vi "压力数据收集.vi"(10 "Value":dbl format="%_3g", 11 "数组in":dbl[][](array[numeric])) -> (1 "添加的数组":dbl[](array[numeric]), 2 "产品型号":string caption="型号字符串", 3 "数组out":dbl[][](array[numeric]))   [LabVIEW 2017]
panel:
  out "添加的数组 19":dbl[](array[numeric])
  out "MAX位置2":dbl
  out "添加的数组 20":dbl[](array[numeric])
  out "MAX位置1":dbl
  out "添加的数组 17":dbl[](array[numeric])
  out "MAX位置3":dbl
  out "添加的数组 18":dbl[](array[numeric])
  out "MAX位置18":dbl
  out "添加的数组 21":dbl[](array[numeric])
  out "MAX位置19":dbl
  out "添加的数组 14":dbl[](array[numeric])
  out "MAX位置17":dbl
  out "添加的数组 15":dbl[](array[numeric])
  out "MAX位置16":dbl
  out "添加的数组 16":dbl[](array[numeric])
  out "MAX位置15":dbl
  out "添加的数组 11":dbl[](array[numeric])
  out "MAX位置14":dbl
  out "添加的数组 12":dbl[](array[numeric])
  out "MAX位置13":dbl
  out "添加的数组 10":dbl[](array[numeric])
  out "MAX位置12":dbl
  out "添加的数组 9":dbl[](array[numeric])
  out "MAX位置11":dbl
  out "添加的数组 8":dbl[](array[numeric])
  out "MAX位置10":dbl
  out "添加的数组 7":dbl[](array[numeric])
  out "MAX位置9":dbl
  out "添加的数组 6":dbl[](array[numeric])
  out "MAX位置8":dbl
  out "添加的数组 5":dbl[](array[numeric])
  out "MAX位置7":dbl
  out "添加的数组 4":dbl[](array[numeric])
  out "MAX位置6":dbl
  out "添加的数组 3":dbl[](array[numeric])
  out "MAX位置5":dbl
  out "添加的数组 2":dbl[](array[numeric])
  out "MAX位置4":dbl
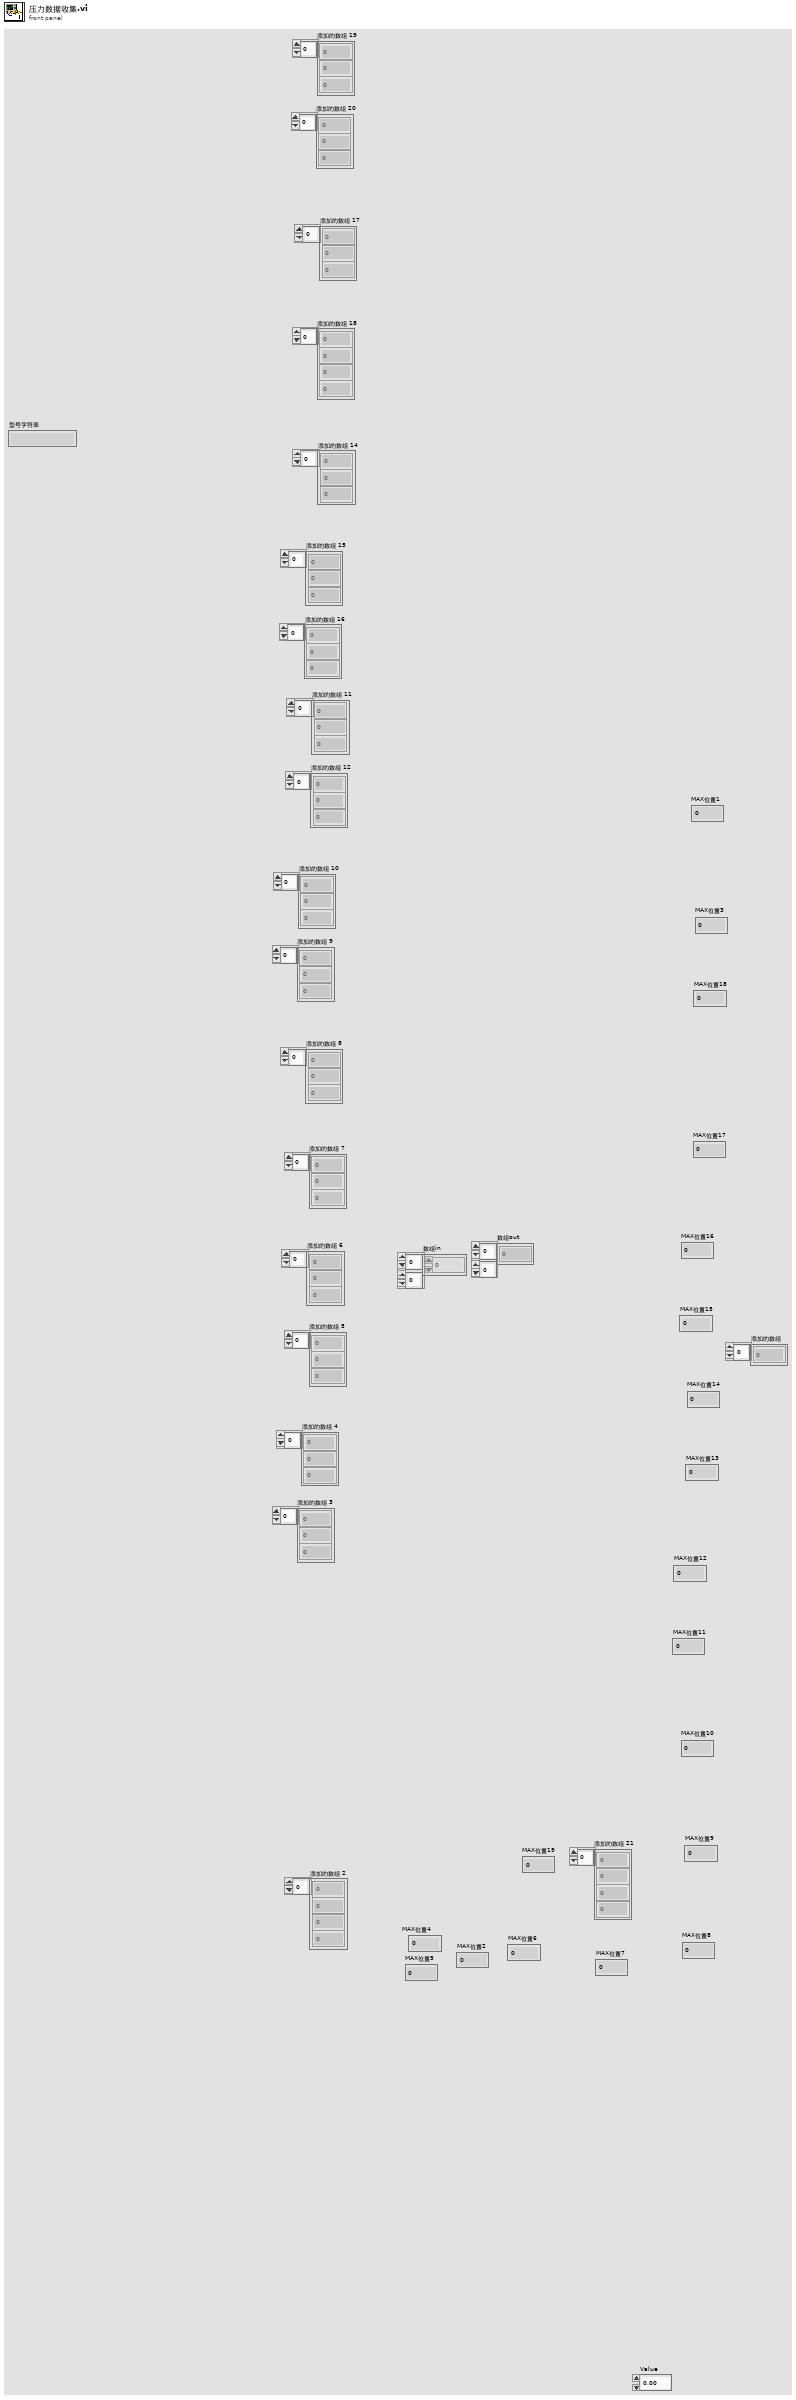
[diagram p1: front panel]
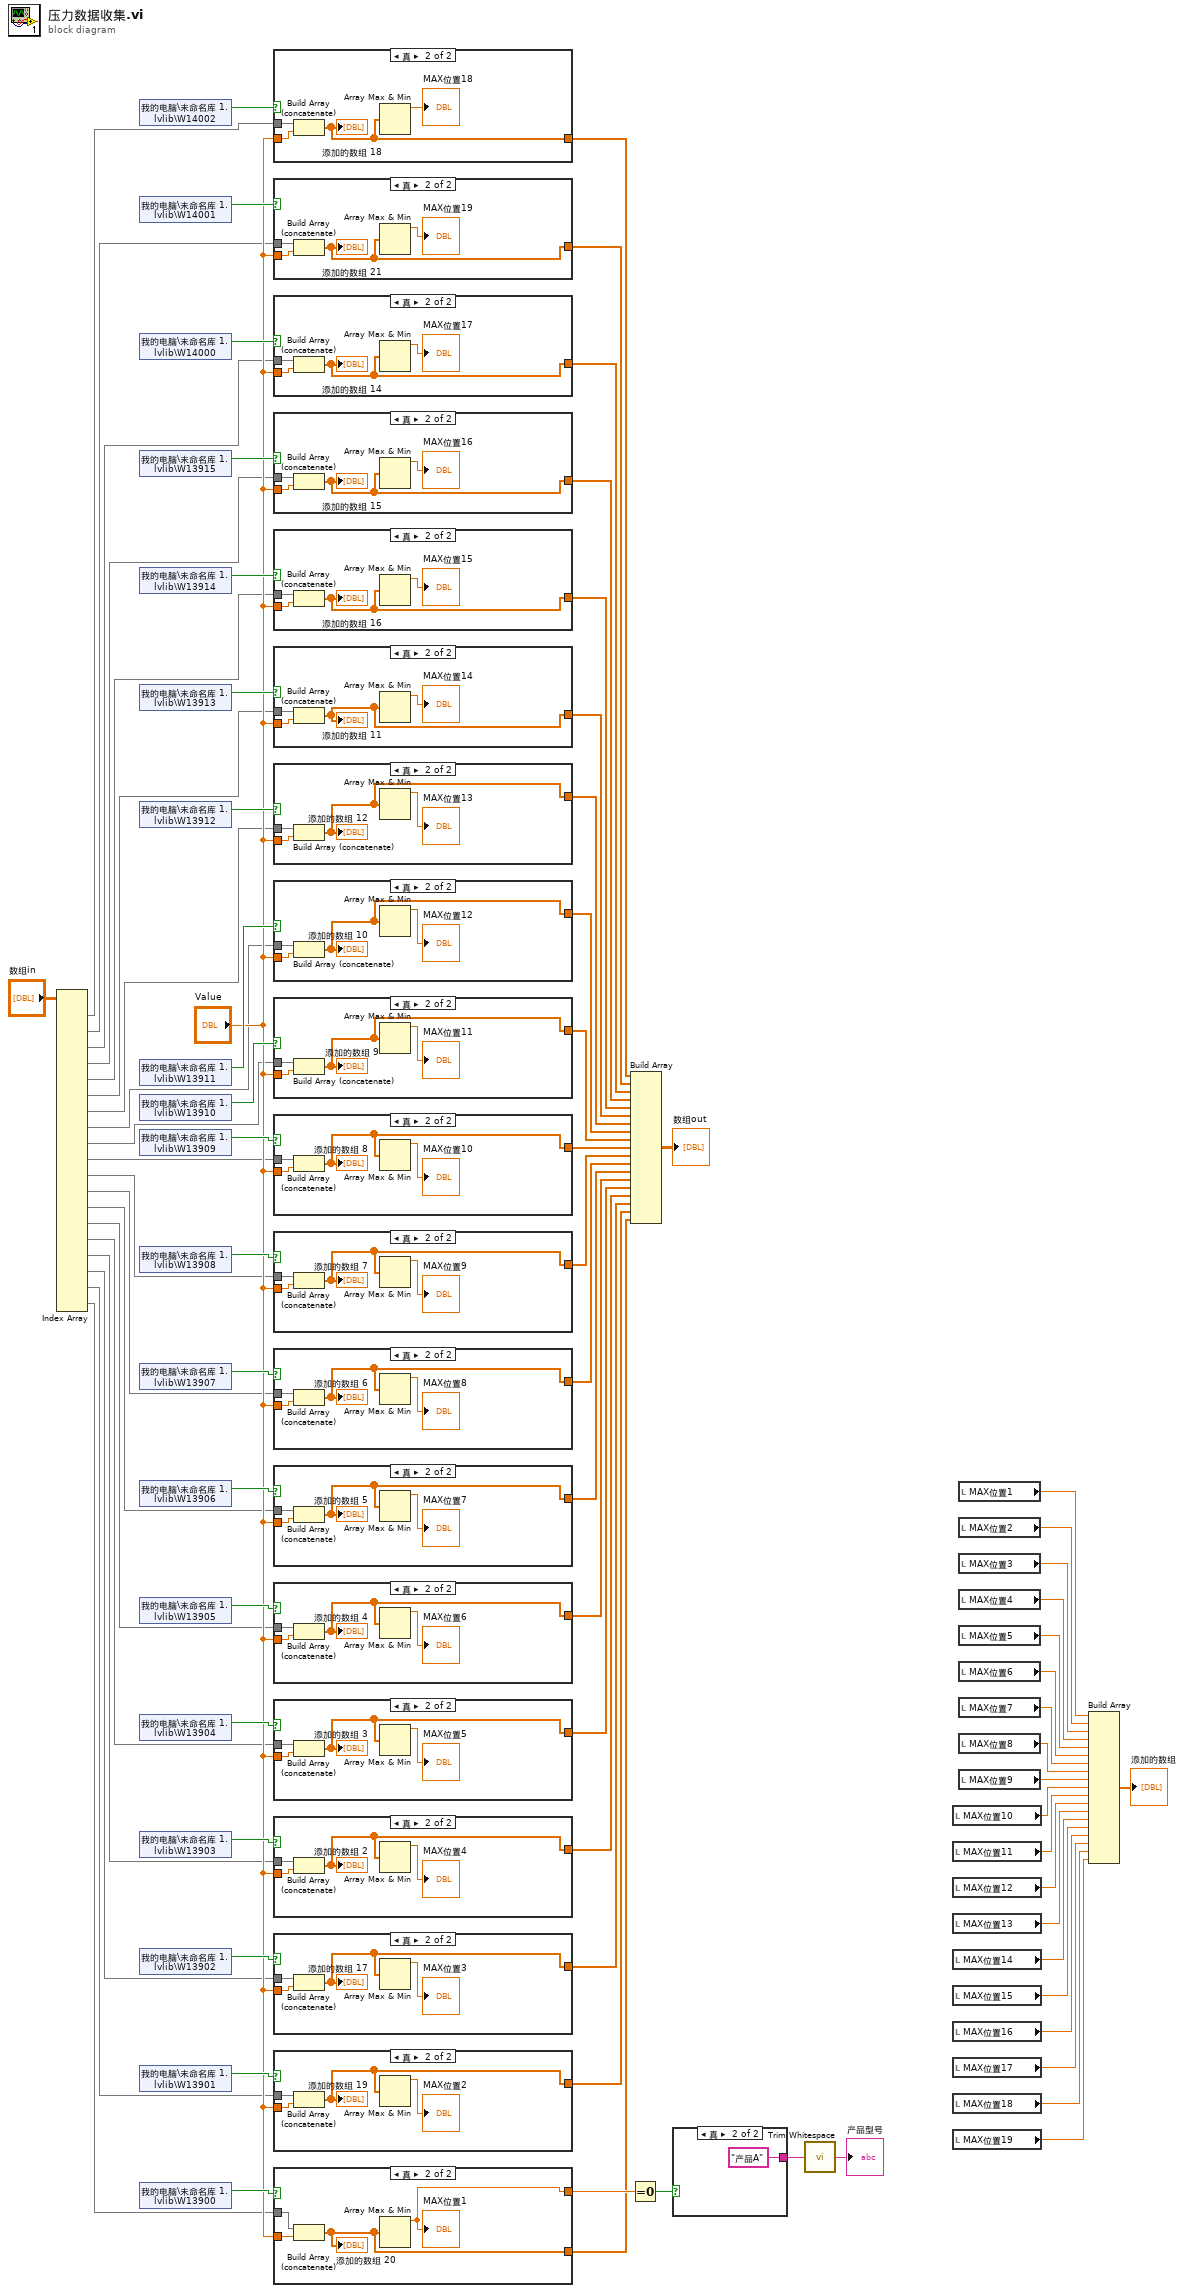
[diagram p0: block diagram]
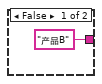
[diagram p2: hidden frame]
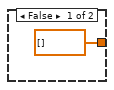
[diagram p3: hidden frame]
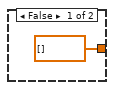
[diagram p4: hidden frame]
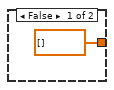
[diagram p5: hidden frame]
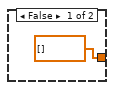
[diagram p6: hidden frame]
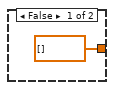
[diagram p7: hidden frame]
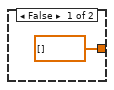
[diagram p8: hidden frame]
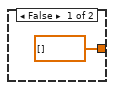
[diagram p9: hidden frame]
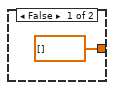
[diagram p10: hidden frame]
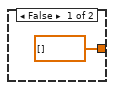
[diagram p11: hidden frame]
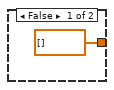
[diagram p12: hidden frame]
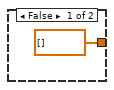
[diagram p13: hidden frame]
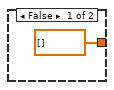
[diagram p14: hidden frame]
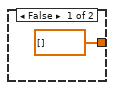
[diagram p15: hidden frame]
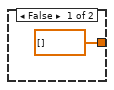
[diagram p16: hidden frame]
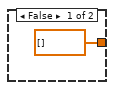
[diagram p17: hidden frame]
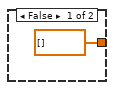
[diagram p18: hidden frame]
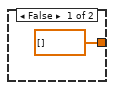
[diagram p19: hidden frame]
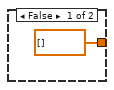
[diagram p20: hidden frame]
diagram:
  n1 = Index Array(array="数组in") -> (element #1=w39:dbl[], element #2=w38:dbl[], element #3=w37:dbl[], element #4=w36:dbl[], element #5=w35:dbl[], element #6=w34:dbl[], element #7=w33:dbl[], element #8=w32:dbl[], element #9=w31:dbl[], element #10=w30:dbl[], element #11=w29:dbl[], element #12=w28:dbl[], element #13=w27:dbl[], element #14=w26:dbl[], element #15=w25:dbl[], element #16=w24:dbl[], element #17=w23:dbl[], element #18=w22:dbl[], element #19=w21:dbl[])  [unwired: 38 in]
  n2 = shared-variable "我的电脑\\未命名库 1.lvlib\\W14002"() -> (w81:bool)  [unwired: 1 in, 1 out]
  n3 = shared-variable "我的电脑\\未命名库 1.lvlib\\W14001"() -> (w66:bool)  [unwired: 1 in, 1 out]
  n4 = shared-variable "我的电脑\\未命名库 1.lvlib\\W14000"() -> (w67:bool)  [unwired: 1 in, 1 out]
  n5 = shared-variable "我的电脑\\未命名库 1.lvlib\\W13915"() -> (w68:bool)  [unwired: 1 in, 1 out]
  n6 = shared-variable "我的电脑\\未命名库 1.lvlib\\W13914"() -> (w69:bool)  [unwired: 1 in, 1 out]
  n7 = shared-variable "我的电脑\\未命名库 1.lvlib\\W13913"() -> (w70:bool)  [unwired: 1 in, 1 out]
  n8 = shared-variable "我的电脑\\未命名库 1.lvlib\\W13912"() -> (w71:bool)  [unwired: 1 in, 1 out]
  n9 = shared-variable "我的电脑\\未命名库 1.lvlib\\W13911"() -> (w72:bool)  [unwired: 1 in, 1 out]
  n10 = shared-variable "我的电脑\\未命名库 1.lvlib\\W13910"() -> (w73:bool)  [unwired: 1 in, 1 out]
  n11 = shared-variable "我的电脑\\未命名库 1.lvlib\\W13909"() -> (w74:bool)  [unwired: 1 in, 1 out]
  n12 = shared-variable "我的电脑\\未命名库 1.lvlib\\W13908"() -> (w75:bool)  [unwired: 1 in, 1 out]
  n13 = shared-variable "我的电脑\\未命名库 1.lvlib\\W13907"() -> (w76:bool)  [unwired: 1 in, 1 out]
  n14 = shared-variable "我的电脑\\未命名库 1.lvlib\\W13906"() -> (w77:bool)  [unwired: 1 in, 1 out]
  n15 = shared-variable "我的电脑\\未命名库 1.lvlib\\W13905"() -> (w78:bool)  [unwired: 1 in, 1 out]
  n16 = shared-variable "我的电脑\\未命名库 1.lvlib\\W13904"() -> (w79:bool)  [unwired: 1 in, 1 out]
  n17 = shared-variable "我的电脑\\未命名库 1.lvlib\\W13903"() -> (w80:bool)  [unwired: 1 in, 1 out]
  n18 = shared-variable "我的电脑\\未命名库 1.lvlib\\W13902"() -> (w83:bool)  [unwired: 1 in, 1 out]
  n19 = shared-variable "我的电脑\\未命名库 1.lvlib\\W13901"() -> (w82:bool)  [unwired: 1 in, 1 out]
  n20 = shared-variable "我的电脑\\未命名库 1.lvlib\\W13900"() -> (w84:bool)  [unwired: 1 in, 1 out]
  n21 = case shown="真" w81 {
    tunnel: [dbl[] [] ("添加的数组") w87] -> w20
    tunnel: "Value" -> [_ w89]
    tunnel: w39 -> [_ w86]
    frame False {
    }
    frame True {
      n22 = Build Array (concatenate)(w86, w89) -> (w87:dbl[])
      "添加的数组 18" <- w87
      n23 = Array Max & Min(array=w87) -> (max value=→"MAX位置18":dbl)  [unwired: 3 out]
    }
  }
  n24 = case shown="真" w66 {
    tunnel: [dbl[] [] ("添加的数组") w92] -> w19
    tunnel: "Value" -> [_ w94]
    tunnel: w38 -> [_ w91]
    frame False {
    }
    frame True {
      n25 = Build Array (concatenate)(w91, w94) -> (w92:dbl[])
      "添加的数组 21" <- w92
      n26 = Array Max & Min(array=w92) -> (max value=→"MAX位置19":dbl)  [unwired: 3 out]
    }
  }
  n27 = case shown="真" w67 {
    tunnel: [dbl[] [] ("添加的数组") w97] -> w18
    tunnel: "Value" -> [_ w99]
    tunnel: w37 -> [_ w96]
    frame False {
    }
    frame True {
      n28 = Build Array (concatenate)(w96, w99) -> (w97:dbl[])
      "添加的数组 14" <- w97
      n29 = Array Max & Min(array=w97) -> (max value=→"MAX位置17":dbl)  [unwired: 3 out]
    }
  }
  n30 = case shown="真" w68 {
    tunnel: [dbl[] [] ("添加的数组") w102] -> w17
    tunnel: "Value" -> [_ w104]
    tunnel: w36 -> [_ w101]
    frame False {
    }
    frame True {
      n31 = Build Array (concatenate)(w101, w104) -> (w102:dbl[])
      "添加的数组 15" <- w102
      n32 = Array Max & Min(array=w102) -> (max value=→"MAX位置16":dbl)  [unwired: 3 out]
    }
  }
  n33 = case shown="真" w69 {
    tunnel: [dbl[] [] ("添加的数组") w107] -> w16
    tunnel: "Value" -> [_ w109]
    tunnel: w35 -> [_ w106]
    frame False {
    }
    frame True {
      n34 = Build Array (concatenate)(w106, w109) -> (w107:dbl[])
      "添加的数组 16" <- w107
      n35 = Array Max & Min(array=w107) -> (max value=→"MAX位置15":dbl)  [unwired: 3 out]
    }
  }
  n36 = case shown="真" w70 {
    tunnel: [dbl[] [] ("添加的数组") w112] -> w15
    tunnel: "Value" -> [_ w114]
    tunnel: w34 -> [_ w111]
    frame False {
    }
    frame True {
      n37 = Build Array (concatenate)(w111, w114) -> (w112:dbl[])
      "添加的数组 11" <- w112
      n38 = Array Max & Min(array=w112) -> (max value=→"MAX位置14":dbl)  [unwired: 3 out]
    }
  }
  n39 = case shown="真" w71 {
    tunnel: [dbl[] [] ("添加的数组") w117] -> w14
    tunnel: "Value" -> [_ w119]
    tunnel: w33 -> [_ w116]
    frame False {
    }
    frame True {
      n40 = Build Array (concatenate)(w116, w119) -> (w117:dbl[])
      "添加的数组 12" <- w117
      n41 = Array Max & Min(array=w117) -> (max value=→"MAX位置13":dbl)  [unwired: 3 out]
    }
  }
  n42 = case shown="真" w72 {
    tunnel: [dbl[] [] ("添加的数组") w122] -> w13
    tunnel: "Value" -> [_ w124]
    tunnel: w32 -> [_ w121]
    frame False {
    }
    frame True {
      n43 = Build Array (concatenate)(w121, w124) -> (w122:dbl[])
      "添加的数组 10" <- w122
      n44 = Array Max & Min(array=w122) -> (max value=→"MAX位置12":dbl)  [unwired: 3 out]
    }
  }
  n45 = case shown="真" w73 {
    tunnel: [dbl[] [] ("添加的数组") w127] -> w12
    tunnel: "Value" -> [_ w129]
    tunnel: w31 -> [_ w126]
    frame False {
    }
    frame True {
      n46 = Build Array (concatenate)(w126, w129) -> (w127:dbl[])
      "添加的数组 9" <- w127
      n47 = Array Max & Min(array=w127) -> (max value=→"MAX位置11":dbl)  [unwired: 3 out]
    }
  }
  n48 = case shown="真" w74 {
    tunnel: [dbl[] [] ("添加的数组") w132] -> w11
    tunnel: "Value" -> [_ w134]
    tunnel: w30 -> [_ w131]
    frame False {
    }
    frame True {
      n49 = Build Array (concatenate)(w131, w134) -> (w132:dbl[])
      "添加的数组 8" <- w132
      n50 = Array Max & Min(array=w132) -> (max value=→"MAX位置10":dbl)  [unwired: 3 out]
    }
  }
  n51 = case shown="真" w75 {
    tunnel: [dbl[] [] ("添加的数组") w137] -> w10
    tunnel: "Value" -> [_ w139]
    tunnel: w29 -> [_ w136]
    frame False {
    }
    frame True {
      n52 = Build Array (concatenate)(w136, w139) -> (w137:dbl[])
      "添加的数组 7" <- w137
      n53 = Array Max & Min(array=w137) -> (max value=→"MAX位置9":dbl)  [unwired: 3 out]
    }
  }
  n54 = case shown="真" w76 {
    tunnel: [dbl[] [] ("添加的数组") w142] -> w9
    tunnel: "Value" -> [_ w144]
    tunnel: w28 -> [_ w141]
    frame False {
    }
    frame True {
      n55 = Build Array (concatenate)(w141, w144) -> (w142:dbl[])
      "添加的数组 6" <- w142
      n56 = Array Max & Min(array=w142) -> (max value=→"MAX位置8":dbl)  [unwired: 3 out]
    }
  }
  n57 = case shown="真" w77 {
    tunnel: [dbl[] [] ("添加的数组") w147] -> w8
    tunnel: "Value" -> [_ w149]
    tunnel: w27 -> [_ w146]
    frame False {
    }
    frame True {
      n58 = Build Array (concatenate)(w146, w149) -> (w147:dbl[])
      "添加的数组 5" <- w147
      n59 = Array Max & Min(array=w147) -> (max value=→"MAX位置7":dbl)  [unwired: 3 out]
    }
  }
  n60 = case shown="真" w78 {
    tunnel: [dbl[] [] ("添加的数组") w152] -> w7
    tunnel: "Value" -> [_ w154]
    tunnel: w26 -> [_ w151]
    frame False {
    }
    frame True {
      n61 = Build Array (concatenate)(w151, w154) -> (w152:dbl[])
      "添加的数组 4" <- w152
      n62 = Array Max & Min(array=w152) -> (max value=→"MAX位置6":dbl)  [unwired: 3 out]
    }
  }
  n63 = case shown="真" w79 {
    tunnel: [dbl[] [] ("添加的数组") w157] -> w6
    tunnel: "Value" -> [_ w159]
    tunnel: w25 -> [_ w156]
    frame False {
    }
    frame True {
      n64 = Build Array (concatenate)(w156, w159) -> (w157:dbl[])
      "添加的数组 3" <- w157
      n65 = Array Max & Min(array=w157) -> (max value=→"MAX位置5":dbl)  [unwired: 3 out]
    }
  }
  n66 = case shown="真" w80 {
    tunnel: [dbl[] [] ("添加的数组") w163] -> w5
    tunnel: "Value" -> [_ w164]
    tunnel: w24 -> [_ w161]
    frame False {
    }
    frame True {
      n67 = Build Array (concatenate)(w161, w164) -> (w163:dbl[])
      "添加的数组 2" <- w163
      n68 = Array Max & Min(array=w163) -> (max value=→"MAX位置4":dbl)  [unwired: 3 out]
    }
  }
  n69 = case shown="真" w83 {
    tunnel: [dbl[] [] ("添加的数组") w167] -> w4
    tunnel: "Value" -> [_ w169]
    tunnel: w23 -> [_ w166]
    frame False {
    }
    frame True {
      n70 = Build Array (concatenate)(w166, w169) -> (w167:dbl[])
      "添加的数组 17" <- w167
      n71 = Array Max & Min(array=w167) -> (max value=→"MAX位置3":dbl)  [unwired: 3 out]
    }
  }
  n72 = case shown="真" w82 {
    tunnel: [dbl[] [] ("添加的数组") w172] -> w3
    tunnel: "Value" -> [_ w174]
    tunnel: w22 -> [_ w171]
    frame False {
    }
    frame True {
      n73 = Build Array (concatenate)(w171, w174) -> (w172:dbl[])
      "添加的数组 19" <- w172
      n74 = Array Max & Min(array=w172) -> (max value=→"MAX位置2":dbl)  [unwired: 3 out]
    }
  }
  n75 = case shown="真" w84 {
    tunnel: [dbl[] [] ("添加的数组") w178] -> w2
    tunnel: "Value" -> [_ w179]
    tunnel: [_ w177] -> w62
    tunnel: w21 -> [_ w176]
    frame False {
    }
    frame True {
      n76 = Build Array (concatenate)(w176, w179) -> (w178:dbl[])
      "添加的数组 20" <- w178
      n77 = Array Max & Min(array=w178) -> (max value=w177:dbl)  [unwired: 3 out]
      "MAX位置1" <- w177
    }
  }
  n78 = Equal To 0?(x=w62) -> (x = 0?=w63:bool)
  n79 = Build Array(w20, w19, w18, w17, w16, w15, w14, w13, w12, w11, w10, w9, w8, w7, w6, w5, w4, w3, w2) -> (→"数组out":dbl[][])
  n80 = case shown="真" w63 {
    tunnel: ["产品B" "产品A"] -> w64
    frame False {
    }
    frame True {
    }
  }
  n81 = call <vilib>:"Trim Whitespace.vi"("string"=w64) -> ("trimmed string"=→"产品型号":string)  [unwired: 1 in]
  n82 = local read "MAX位置10"() -> (w51:dbl)
  n83 = local read "MAX位置11"() -> (w50:dbl)
  n84 = local read "MAX位置12"() -> (w49:dbl)
  n85 = local read "MAX位置13"() -> (w48:dbl)
  n86 = local read "MAX位置14"() -> (w47:dbl)
  n87 = local read "MAX位置15"() -> (w46:dbl)
  n88 = local read "MAX位置16"() -> (w45:dbl)
  n89 = local read "MAX位置17"() -> (w44:dbl)
  n90 = local read "MAX位置18"() -> (w43:dbl)
  n91 = local read "MAX位置19"() -> (w42:dbl)
  n92 = local read "MAX位置1"() -> (w60:dbl)
  n93 = local read "MAX位置2"() -> (w59:dbl)
  n94 = local read "MAX位置3"() -> (w58:dbl)
  n95 = local read "MAX位置4"() -> (w57:dbl)
  n96 = local read "MAX位置5"() -> (w56:dbl)
  n97 = local read "MAX位置6"() -> (w55:dbl)
  n98 = local read "MAX位置7"() -> (w54:dbl)
  n99 = local read "MAX位置8"() -> (w53:dbl)
  n100 = local read "MAX位置9"() -> (w52:dbl)
  n101 = Build Array(w60, w59, w58, w57, w56, w55, w54, w53, w52, w51, w50, w49, w48, w47, w46, w45, w44, w43, w42) -> (→"添加的数组":dbl[])
